vi "Example Callback.vi"() -> ()   [LabVIEW 2010]
uses:
  C:/tf/play/labview/Tinkerforge.dll
panel:
  out "detection cycle ended counter":i32
  in  "stop":bool
  out "motion detected counter":i32
  in  "uid":string="gtr"
  in  "port":i32=4223
  in  "host":string="localhost"
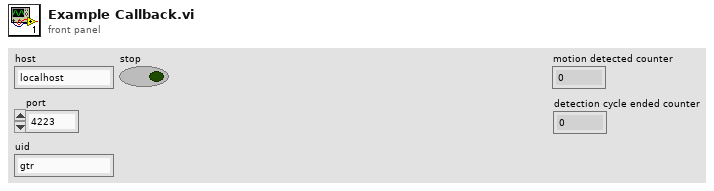
[diagram p1: front panel]
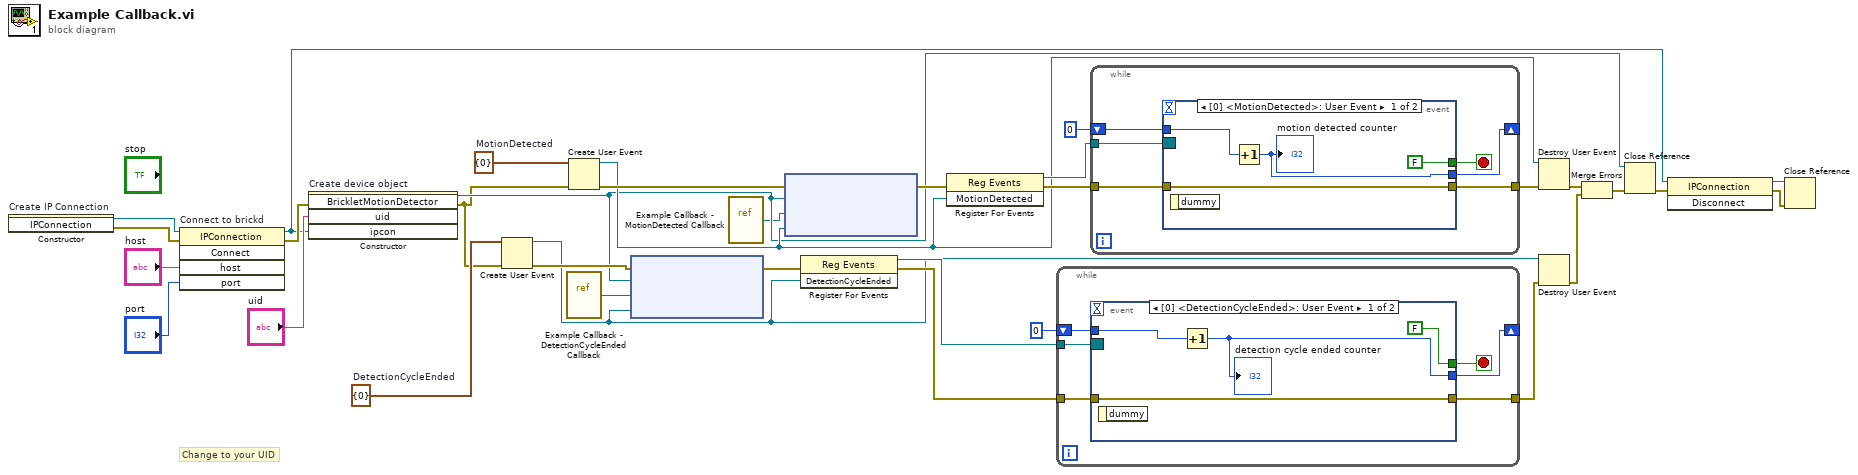
[diagram p0: block diagram]
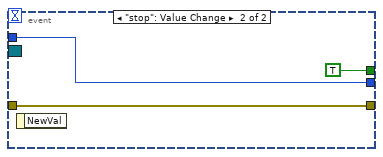
[diagram p2: hidden frame]
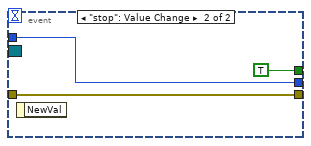
[diagram p3: hidden frame]
diagram:
  w7 = cluster{"dummy":u8} {"dummy"=0}  # DetectionCycleEnded
  w18 = cluster{"dummy":u8} {"dummy"=0}  # MotionDetected
  # "Change to your UID"
  n1 = constructor on="Create IP Connection" class="IPConnection"() -> (reference out=w33:refnum<k24>, error out=w5:errorcluster)  [unwired: 3 in, 1 out]
  n2 = invoke on="Connect to brickd" class="IPConnection" method="Connect"(reference=w33, error in=w5, "host"="host", "port"="port") -> (reference out=w26:refnum<k24>, error out=w29:errorcluster)  [unwired: 1 in, 3 out]
  n3 = constructor on="Create device object" class="BrickletMotionDetector"(error in=w29, "uid"="uid", "ipcon"=w26) -> (reference out=w8:refnum<k24>, error out=w6:errorcluster)  [unwired: 2 in, 3 out]
  n4 = Create User Event(user event datatype=w7, error in=w6) -> (user event=w10:refnum<user-event>, error out=w15:errorcluster)
  n5 = vi-ref "Example Callback - DetectionCycleEnded Callback.vi"() -> ("vi reference"=w1:refnum<vi>)
  n6 = Create User Event(user event datatype=w18, error in=w6) -> (user event=w19:refnum<user-event>, error out=w24:errorcluster)
  n7 = node ("Register Event Callback")(w15, w8, w1, w10) -> (w14:errorcluster)  [unwired: 1 in, 1 out]
  n8 = vi-ref "Example Callback - MotionDetected Callback.vi"() -> ("vi reference"=w2:refnum<vi>)
  n9 = node ("Register Event Callback")(w24, w8, w2, w19) -> (w23:errorcluster)  [unwired: 1 in, 1 out]
  n10 = register-events(error in=w14, w10) -> (reference out=w13:refnum<event-registration>, error out=w11:errorcluster)  [unwired: 1 in]
  n11 = register-events(error in=w23, w19) -> (reference out=w22:refnum<event-registration>, error out=w20:errorcluster)  [unwired: 1 in]
  n12 = while {
    tunnel: w13 -> [w39]
    tunnel: [w38] -> w12
    tunnel: w11 -> [w37]
    shift-right: [w34] -> _
    shift-left: 0 -> [w35]
    stop <- w36 stop-if-true
    n13 = event shown="[0] <DetectionCycleEnded>: User Event" {
      selector: w39 -> [_ _]
      dyn-events: _ -> [_ _]
      timeout: _ -> [_ _]
      tunnel: [w43 w45] -> w38
      tunnel: w37 -> [w43 w45]
      tunnel: [FALSE TRUE] -> w36
      tunnel: w35 -> [w41 w44]
      tunnel: [w40 w44] -> w34
      event User Event {
        n14 = event-data() -> ()  [unwired: 1 in, 1 out]
        n15 = Increment(x=w41) -> (x+1=w40:i32)
        "detection cycle ended counter" <- w40
      }
      event "stop": Value Change {
        n16 = event-data() -> ()  [unwired: 1 in, 1 out]
      }
    }
  }
  n17 = while {
    tunnel: w22 -> [w52]
    tunnel: [w51] -> w21
    tunnel: w20 -> [w50]
    shift-right: [w47] -> _
    shift-left: 0 -> [w48]
    stop <- w49 stop-if-true
    n18 = event shown="[0] <MotionDetected>: User Event" {
      selector: w52 -> [_ _]
      dyn-events: _ -> [_ _]
      timeout: _ -> [_ _]
      tunnel: [w56 w58] -> w51
      tunnel: w50 -> [w56 w58]
      tunnel: [FALSE TRUE] -> w49
      tunnel: w48 -> [w54 w57]
      tunnel: [w53 w57] -> w47
      event User Event {
        n19 = event-data() -> ()  [unwired: 1 in, 1 out]
        n20 = Increment(x=w54) -> (x+1=w53:i32)
        "motion detected counter" <- w53
      }
      event "stop": Value Change {
        n21 = event-data() -> ()  [unwired: 1 in, 1 out]
      }
    }
  }
  n22 = Destroy User Event(user event=w19, error in=w21) -> (error out=w17:errorcluster)
  n23 = Destroy User Event(user event=w10, error in=w12) -> (error out=w9:errorcluster)
  n24 = Merge Errors(w17, w9) -> (w16:errorcluster)
  n25 = Close Reference(reference=w8, error in (no error)=w16) -> (error out=w28:errorcluster)
  n26 = invoke class="IPConnection" method="Disconnect"(reference=w26, error in=w28) -> (reference out=w25:refnum<k24>, error out=w27:errorcluster)  [unwired: 1 in, 1 out]
  n27 = Close Reference(reference=w25, error in (no error)=w27) -> ()  [unwired: 1 out]
